vi "Commanded stage name available.vi"(0 "System no.":i32=1 min=1 max=4 step=1, 2 "Commanded stages":string[](array[string]), 5 "error in":errorcluster) -> (14 "Controller error":bool, 19 "error out":errorcluster)   [LabVIEW 2026]
doc: "This VI checks if Commanded stages is a subset of all available stages and returns Controller error TRUE if this is not the case. Available stages are defined by VST?.vi."
panel:
  out "Available stages":string[](array[string])
  # "This VI checks if \"Commanded stages\" is a subset of all available stages and returns \"Controller error\" TRUE if this is not the case. Available stages are defined by VST?.vi."
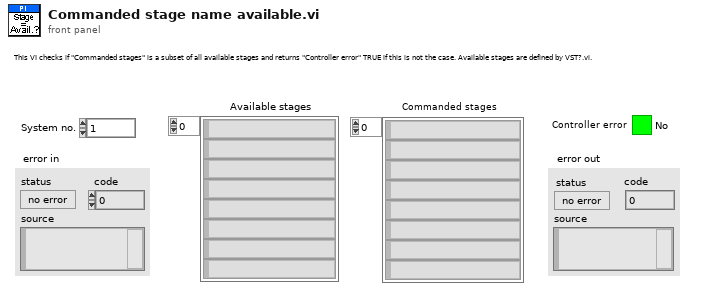
[diagram p1: front panel]
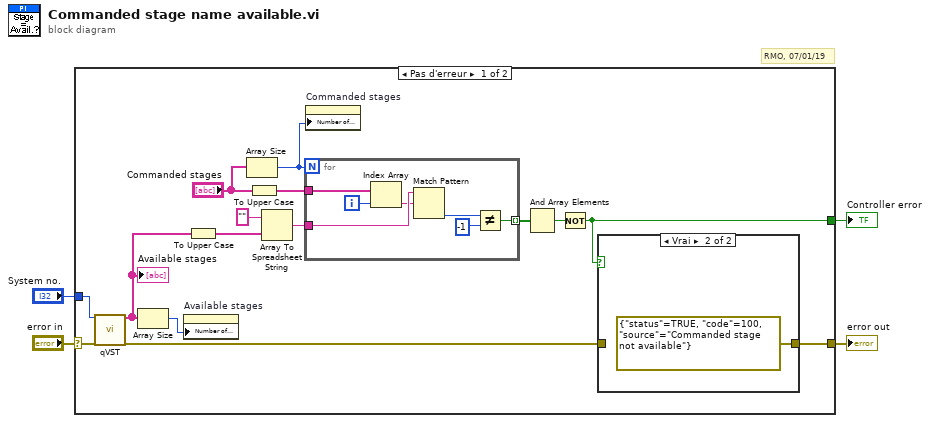
[diagram p0: block diagram]
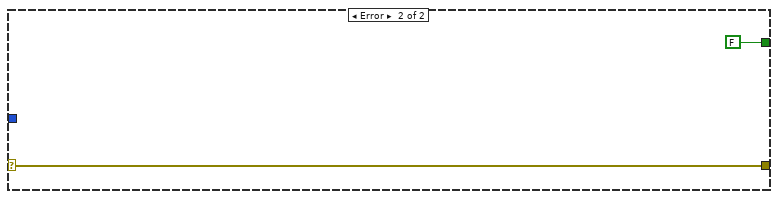
[diagram p3: hidden frame]
diagram:
  # "RMO, 07/01/19"
  n1 = case shown="Pas d'erreur" "error in" {
    selector: "error in" -> [w6 w30]
    tunnel: [w13 w30] -> w4
    tunnel: "System no." -> [w7 _]
    tunnel: [w5 FALSE] -> w1
    frame No Error {
      n2 = call "qVST.vi"("System no."=w7, "error in"=w6) -> ("Available stages"=w8:string[], "error out"=w9:errorcluster)  [unwired: 16 out]
      "Available stages" <- w8
      n3 = Array Size(array=w8) -> (size(s)=w11:i32)
      n4 = property on="Available stages" class="Tabl (strict)"("Number of Rows"=w11) -> ()  [unwired: 2 in, 2 out]
      n5 = To Upper Case(1:w8) -> (0:w10:string[])
      n6 = Array Size(array="Commanded stages") -> (size(s)=w12:i32)
      n7 = To Upper Case(1:"Commanded stages") -> (0:w15:string[])
      n8 = Array To Spreadsheet String(array=w10, 3:"" ("format string")) -> (spreadsheet string=w19:string)  [unwired: 1 out]
      n9 = for {
        N: w12 -> [_]
        tunnel: w19 -> [w28]
        tunnel: w15 -> [w27]
        tunnel: [w22] -> w18 mode=indexing
        i -> [w26]
        n10 = Index Array(array=w27, index=w26) -> (element=w25:string)
        n11 = Match Pattern(string=w28, regular expression=w25) -> (offset past match=w23:i32)  [unwired: 4 out]
        n12 = Not Equal?(x=w23, y=-1) -> (x != y?=w22:bool)
      }
      n13 = property on="Commanded stages" class="Tabl (strict)"("Number of Rows"=w12) -> ()  [unwired: 2 in, 2 out]
      n14 = And Array Elements(Boolean array=w18) -> (logical AND=w17:bool)
      n15 = Not(x=w17) -> (.not. x?=w5:bool)
      n16 = case shown="Vrai" w5 {
        tunnel: [w20 errorcluster {"status"=TRUE, "code"=100, "source"="Commanded stage not available"} ("error out")] -> w13
        tunnel: w9 -> [w20 _]
        frame False {
        }
        frame True {
        }
      }
    }
    frame Error {
    }
  }
  "error out" <- w4
  "Controller error" <- w1
